vi "Cool Until Target.vi"(8 "error in (no error)":errorcluster, 10 "target temperature":dbl[unit]=273.15, 11 "cooling system in":refnum<class "Evaporative Cooler.lvclass">) -> (0 "error out":errorcluster, 3 "cooling system out":refnum<class "Evaporative Cooler.lvclass">)   [LabVIEW 2023, in "Evaporative Cooler.lvclass"]
uses:
  Evaporative Cooler.lvclass
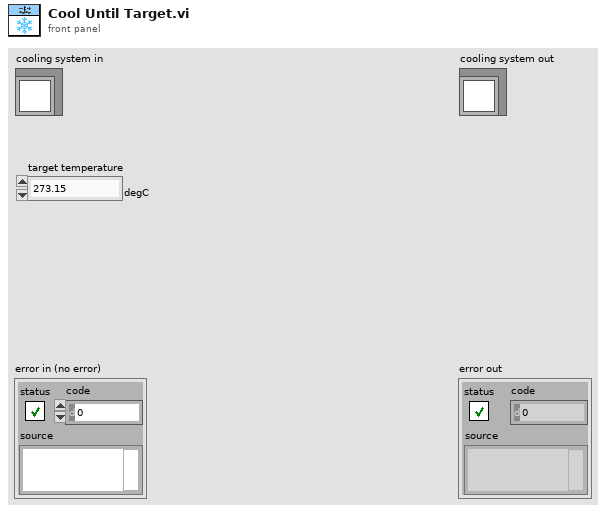
[diagram p1: front panel]
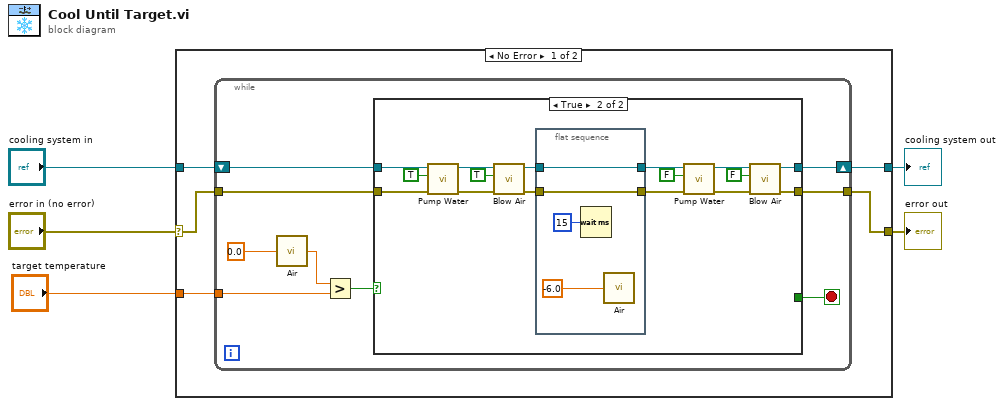
[diagram p0: block diagram]
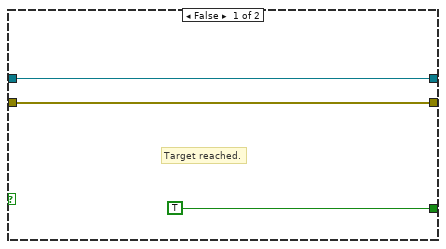
[diagram p2: hidden frame]
diagram:
  n1 = case shown="No Error" "error in (no error)" {
    selector: "error in (no error)" -> [w8 w44]
    tunnel: "target temperature" -> [w10 _]
    tunnel: [w7 w44] -> w3
    tunnel: "cooling system in" -> [w9 w43]
    tunnel: [w6 w43] -> w1
    frame No Error {
      n2 = while {
        tunnel: w10 -> [w18]
        tunnel: w8 -> [w13]
        tunnel: [w12] -> w7
        shift-right: [w11] -> w6
        shift-left: w9 -> [w14]
        stop <- w15 stop-if-true
        n3 = call "Air.vi"("temperature adjustment"=dbl[unit] 0.0) -> ("new air temperature"=w17:dbl[unit])
        n4 = Greater?(x=w17, y=w18) -> (0:w16:bool)
        n5 = case shown="True" w16 {
          tunnel: [TRUE _] -> w15
          tunnel: w14 -> [w21 w37]
          tunnel: w13 -> [w20 w25]
          tunnel: [w20 w24] -> w12
          tunnel: [w21 w23] -> w11
          frame False {
            # "Target reached."
          }
          frame True {
            n6 = call "Pump Water.vi"("error in (no error)"=w25, "enable?"=TRUE, "Swamp Cooler in"=w37) -> ("error out"=w36:errorcluster, "Swamp Cooler out"=w35:refnum<class "Evaporative Cooler.lvclass">)  [unwired: 7 in]
            n7 = call "Blow Air.vi"("error in (no error)"=w36, "enable?"=TRUE, "Swamp Cooler in"=w35) -> ("error out"=w32:errorcluster, "Swamp Cooler out"=w33:refnum<class "Evaporative Cooler.lvclass">)  [unwired: 7 in]
            n8 = flat-sequence {
              tunnel: [w41] -> w27
              tunnel: w33 -> [w41]
              tunnel: [w40] -> w26
              tunnel: w32 -> [w40]
              frame #0 {
                n9 = Wait (ms)(milliseconds to wait=u32 15) -> ()  [unwired: 1 out]
                n10 = call "Air.vi"("temperature adjustment"=dbl[unit] -6.0) -> ()  [unwired: 1 out]
              }
            }
            n11 = call "Pump Water.vi"("error in (no error)"=w26, "enable?"=FALSE, "Swamp Cooler in"=w27) -> ("error out"=w29:errorcluster, "Swamp Cooler out"=w30:refnum<class "Evaporative Cooler.lvclass">)  [unwired: 7 in]
            n12 = call "Blow Air.vi"("error in (no error)"=w29, "enable?"=FALSE, "Swamp Cooler in"=w30) -> ("error out"=w24:errorcluster, "Swamp Cooler out"=w23:refnum<class "Evaporative Cooler.lvclass">)  [unwired: 7 in]
          }
        }
      }
    }
    frame Error {
    }
  }
  "error out" <- w3
  "cooling system out" <- w1
